vi "VScaleVals.vi"(11 "Full Scale":dbl) -> (1 "vGain (dB)":dbl, 2 "Total Gain (dB)":dbl, 3 "Voltage Scale":T1)   [LabVIEW 2022 SP3]
uses:
  Pulsers/PulserGlobals.vi
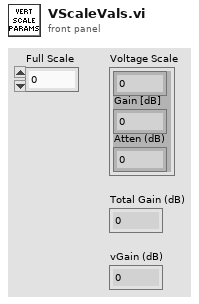
[diagram p1: front panel]
types:
  T1 = cluster{sgl, "Gain [dB]  ":sgl, "Atten (dB)":sgl}
  T2 = typedef "pulser.ctl" = enum16{"Pan 5900", "Daxsonics", "Agilent 33xxx", "UTEX", "JSR", "WMC Mono-Cycle", "No Pulser", "NYU AVTECH", "Tabor W1281A", "Pan 5800", "Unlisted", "Tabor WX2182B"}
  T3 = cluster{"Energy (microJ)":u8, "Damping (In Ohm)":u8, "HP Filt(KHz) ":u16, "LP Filt (MHz)":u8, "Gain (db)":u8, "Atten (dB)":sgl}
  T4 = cluster{"Full Scale":dbl, "Gain [dB]  ":sgl, "Atten (dB)":sgl}
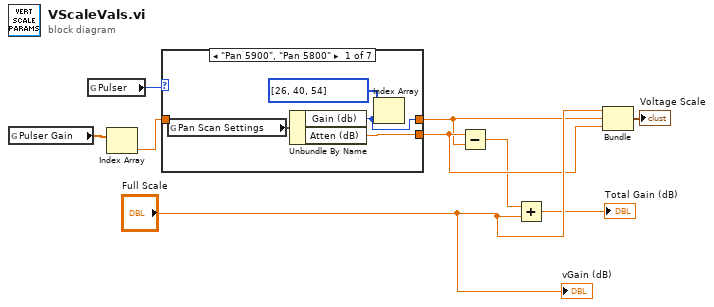
[diagram p0: block diagram]
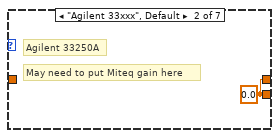
[diagram p2: hidden frame]
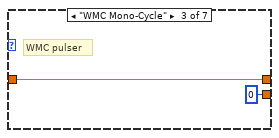
[diagram p3: hidden frame]
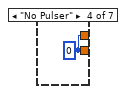
[diagram p4: hidden frame]
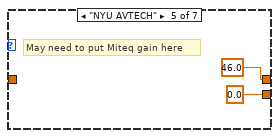
[diagram p5: hidden frame]
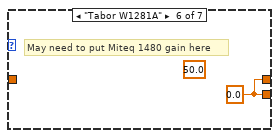
[diagram p6: hidden frame]
diagram:
  n1 = global read "PulserGlobals.vi" "Pulser Gain"() -> (w2:sgl[])
  n2 = global read "PulserGlobals.vi" "Pulser"() -> (w1:T2)
  n3 = Index Array(array=w2) -> (element=w3:sgl)  [unwired: 1 in]
  n4 = case shown="\"Pan 5900\", \"Pan 5800\"" w1 {
    tunnel: [w12 w14 0 w17 sgl 0.0 w20 _] -> w8
    tunnel: [w11 w14 w15 w17 sgl 46.0 w20 w21] -> w7
    tunnel: w3 -> [_ _ w15 _ _ _ w21]
    frame "Pan 5900", "Pan 5800" {
      n5 = global read "PulserGlobals.vi" "Pan Scan Settings"() -> (w10:T3)
      n6 = Unbundle By Name(w10) -> ("Gain (db)"=w11:u8, "Atten (dB)"=w12:sgl)
      n7 = Index Array(array=i32[] [26, 40, 54], index=w11) -> ()  [unwired: 1 out]
    }
    frame "Agilent 33xxx", Default {
      w14 = sgl 0.0
      # "Agilent 33250A"
      # "May need to put Miteq gain here"
    }
    frame "WMC Mono-Cycle" {
      # "WMC pulser"
    }
    frame "No Pulser" {
      w17 = 0
    }
    frame "NYU AVTECH" {
      # "May need to put Miteq gain here"
    }
    frame "Tabor W1281A" {
      (unwired) sgl 50.0
      w20 = sgl 0.0
      # "May need to put Miteq 1480 gain here"
    }
    frame "Daxsonics" {
    }
  }
  n8 = Subtract(x=w8, y=w7) -> (x-y=w5:sgl)
  n9 = Add(x=w5, y="Full Scale") -> (x+y=→"Total Gain (dB)":dbl)
  n10 = Bundle("Full Scale"="Full Scale", "Gain [dB]"=w7, "Atten (dB)"=w8) -> (→"Voltage Scale":T4)  [unwired: 1 out]
  "vGain (dB)" <- "Full Scale"
